vi "ProyectoFinal.vi"() -> ()   [LabVIEW 2020]
uses:
  <vilib>/Instr/_visa.llb/VISA Configure Serial Port (Instr).vi
  <vilib>/addons/control/pid/pid.llb/PID (DBL).vi
  <vilib>/addons/control/pid/NI_PID_pid.lvlib
panel:
  out "Thermometer A":dbl(slide) scale=0.0..32.0
  in  "MANUAL / MATERIAL":bool
  in  "LISTA DE MATERIALES":string(combo)
  out "Temp Reci 2":dbl
  out "Temp Reci":dbl
  in  "EXTRUIR":bool
  out "PRECALENTADO":bool
  in  "Set Point":dbl(slide) scale=0.0..40.0
  out "Temp Fil 2":dbl
  out "ERROR 2":dbl
  out "ErrorPID 2":dbl
  out "Error PID 2":dynamicdata(graph)
  out "Temperatura 2":dynamicdata(graph)
  out "Error PID":dynamicdata(graph)
  in  "VISA resource name":refnum<visa-resource-name>
  in  "stop":bool
  out "ERROR":dbl
  out "Temperatura":dynamicdata(graph)
  out "Temp Fil":dbl
  out "ErrorPID":dbl
  # "CONTROLADOR SISTEMA TERMICO CON CONTROL PID COMUNICACION SERIE"
  # "UNIDAD PROFESIONAL DE INGENIERIA CAMPUS ZACATECAS - INSTITUTO POLITECNICO NACIONAL\nUNIDAD DE APREDIZAJE DE INSTRUMENTACION VIRTUAL\nDIEGO JAUREGUI ONTIVEROS  | CARLOS CASAS CASAS | ALEJANDRO LOPEZ GONZALEZ"
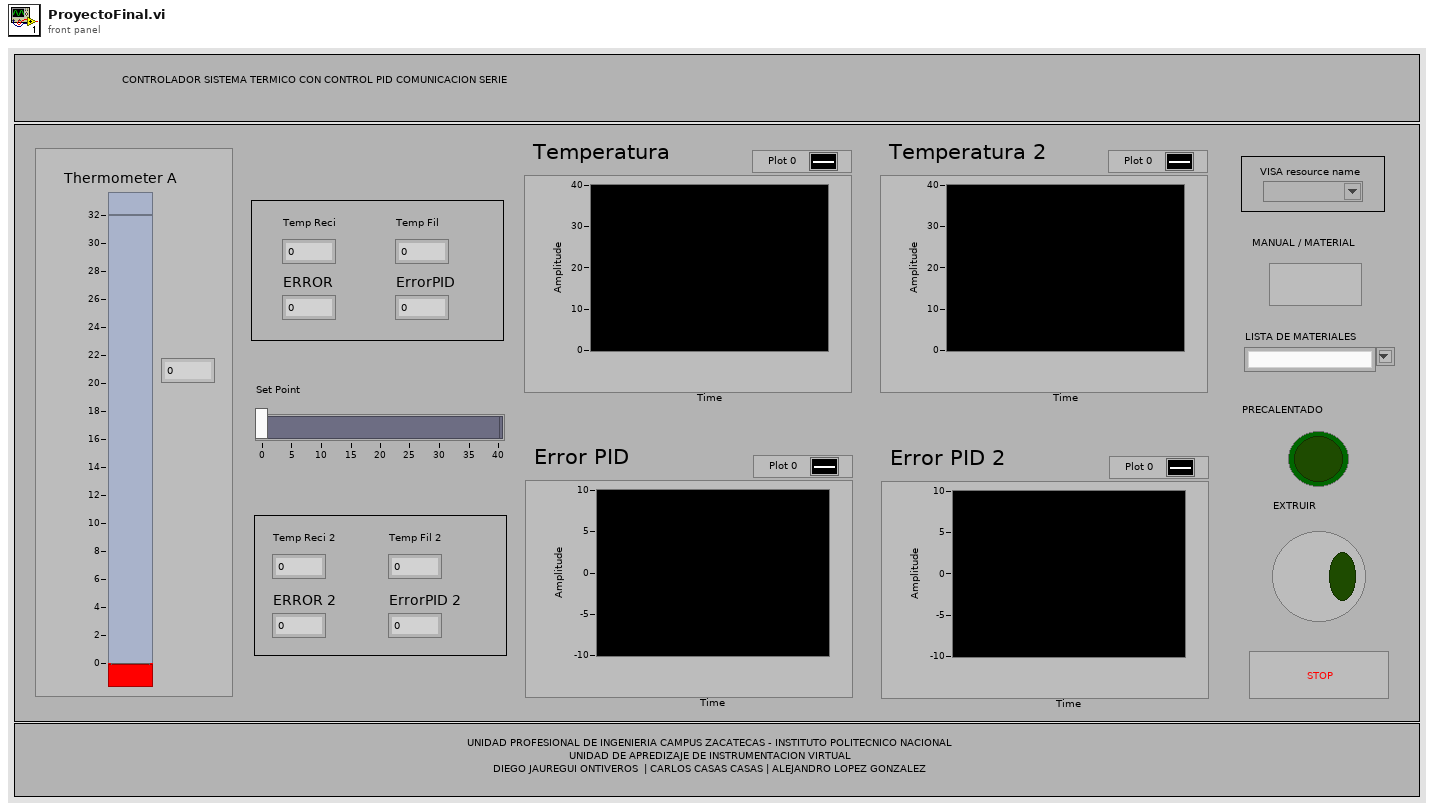
[diagram p1: front panel]
types:
  T1 = cluster{"proportional gain (Kc)":dbl, "integral time (Ti, min)":dbl, "derivative time (Td, min)":dbl}
  T2 = enum8{"Enabled", "Disabled", "Disabled and Grayed Out"}
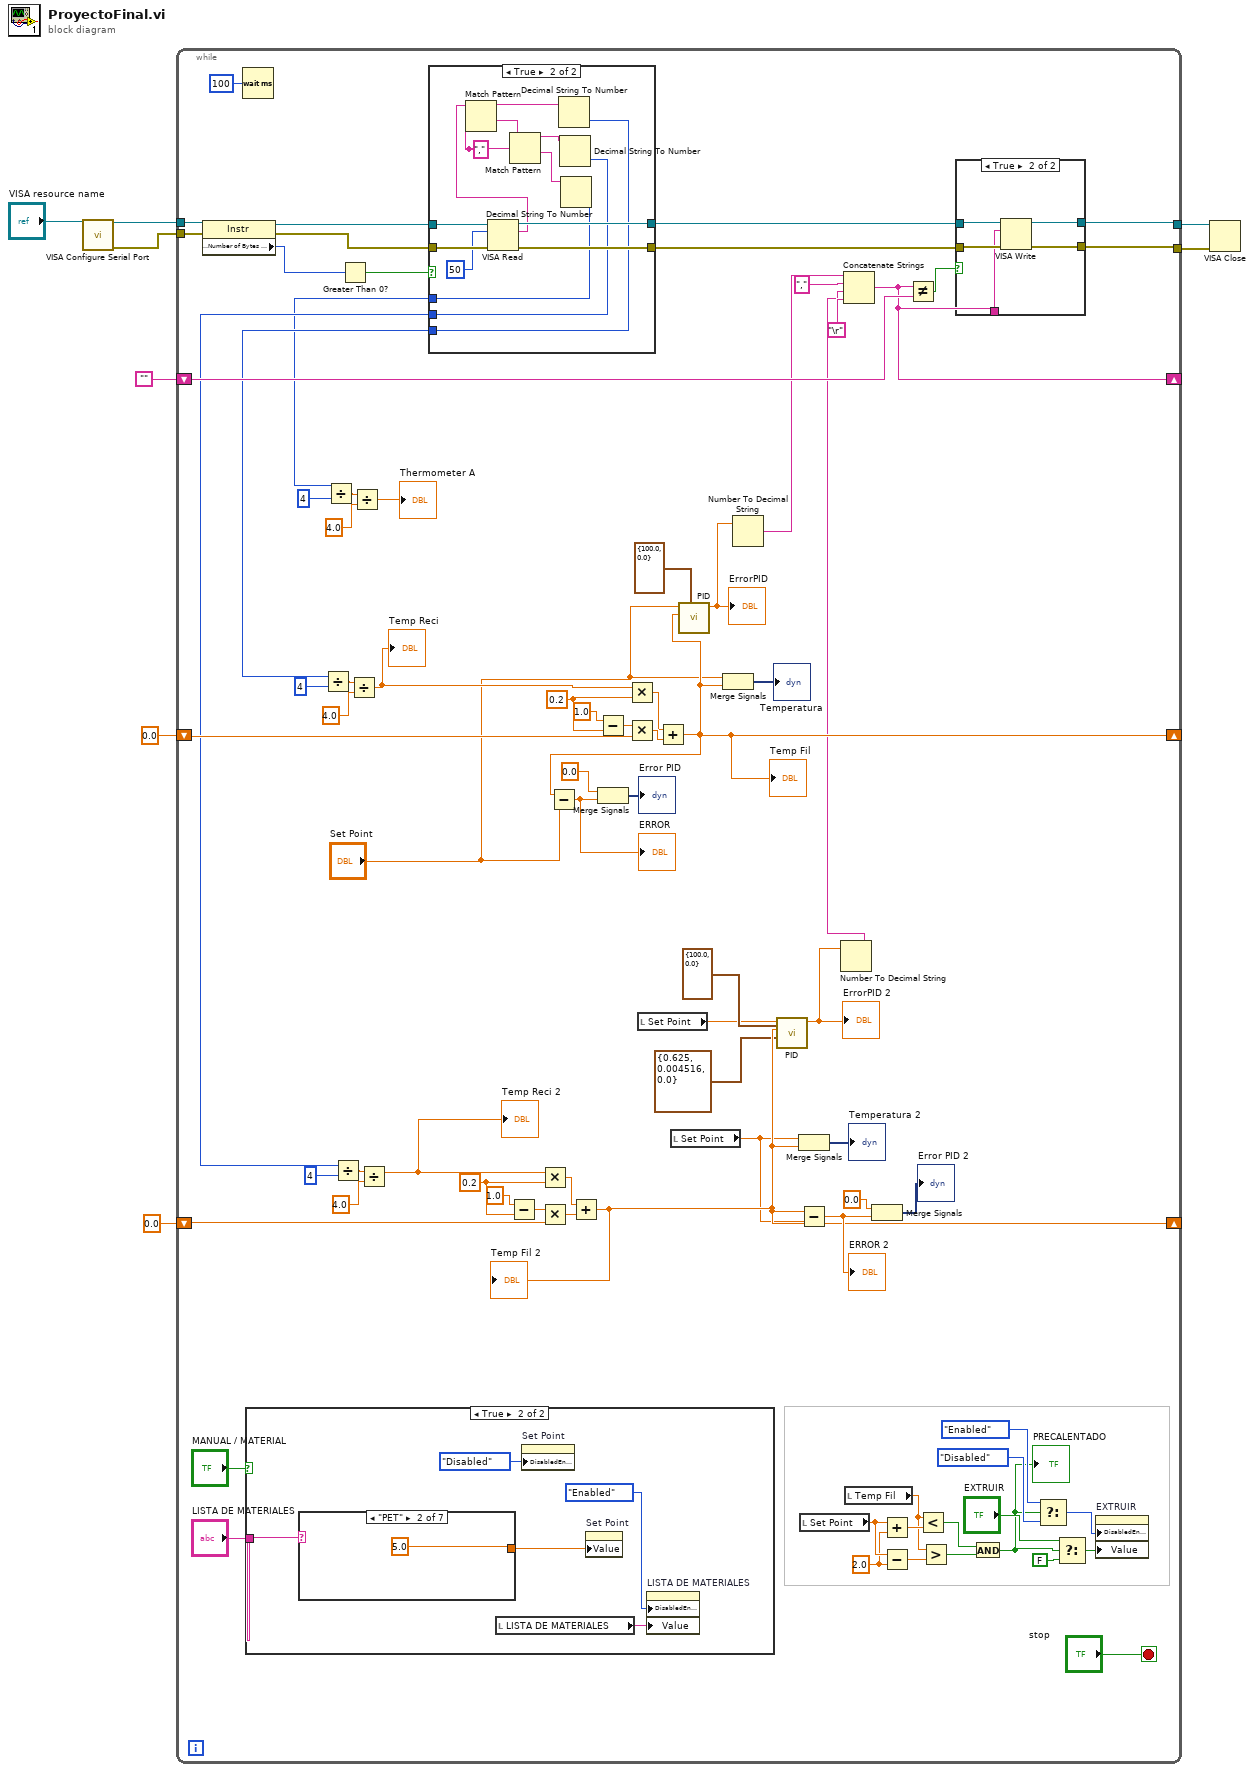
[diagram p0: block diagram]
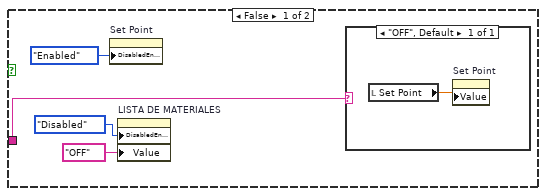
[diagram p2: hidden frame]
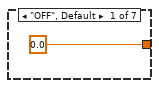
[diagram p3: hidden frame]
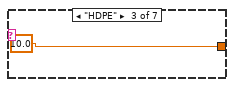
[diagram p4: hidden frame]
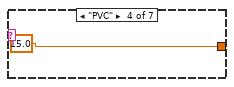
[diagram p5: hidden frame]
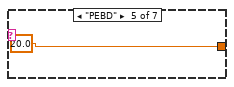
[diagram p6: hidden frame]
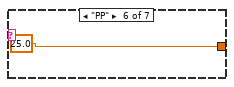
[diagram p7: hidden frame]
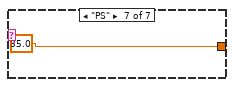
[diagram p8: hidden frame]
diagram:
  n1 = call-poly "VISA Configure Serial Port"("VISA resource name"="VISA resource name") -> ("VISA resource name out"=w6:refnum<visa-resource-name>, "error out"=w5:errorcluster)  [unwired: 13 in]
  n2 = while {
    tunnel: [w87] -> w8
    tunnel: [w86] -> w7
    tunnel: w6 -> [w85]
    tunnel: w5 -> [w84]
    shift-right: [w82] -> _
    shift-left: "" -> [w83]
    shift-right: [w44] -> _
    shift-left: 0.0 -> [w66]
    shift-right: [w12] -> _
    shift-left: 0.0 -> [w49]
    stop <- "stop" stop-if-true
    w29 = 2.0 ("y")
    w52 = 0.2
    w68 = 0.2
    n3 = property class="Instr"(reference=w85, error in=w84) -> (reference out=w80:refnum<visa-resource-name>, error out=w78:errorcluster, "Serial Settings:Number of Bytes at Serial Port"=w75:u32)
    n4 = Wait (ms)(milliseconds to wait=u32 100) -> ()  [unwired: 1 out]
    n5 = case shown="True" "MANUAL / MATERIAL" {
      tunnel: "LISTA DE MATERIALES" -> [w89 w95]
      frame False {
        n6 = property on="Set Point" class="Slide (strict)"("DisabledEnum"=T2."Enabled" ("Disabled")) -> ()  [unwired: 2 in, 2 out]
        n7 = property on="LISTA DE MATERIALES" class="CmbBox"("DisabledEnum"=T2."Disabled" ("Disabled"), "Value"="OFF" ("LISTA DE MATERIALES")) -> ()  [unwired: 2 in, 2 out]
        n8 = case shown="\"OFF\", Default" w89 {
          frame "OFF", Default {
            n9 = local read "Set Point"() -> (w93:dbl)
            n10 = property on="Set Point" class="Slide (strict)"("Value"=w93) -> ()  [unwired: 2 in, 2 out]
          }
        }
      }
      frame True {
        n11 = case shown="\"PET\"" w95 {
          tunnel: [0.0 ("Set Point") 5.0 ("Set Point") 10.0 ("Set Point") 15.0 ("Set Point") 20.0 ("Set Point") 25.0 ("Set Point") 35.0 ("Set Point")] -> w94
          frame "OFF", Default {
          }
          frame "PET" {
          }
          frame "HDPE" {
          }
          frame "PVC" {
          }
          frame "PEBD" {
          }
          frame "PP" {
          }
          frame "PS" {
          }
        }
        n12 = local read "LISTA DE MATERIALES"() -> (w96:string)
        n13 = property on="Set Point" class="Slide (strict)"("DisabledEnum"=T2."Disabled" ("Disabled")) -> ()  [unwired: 2 in, 2 out]
        n14 = property on="Set Point" class="Slide (strict)"("Value"=w94) -> ()  [unwired: 2 in, 2 out]
        n15 = property on="LISTA DE MATERIALES" class="CmbBox"("DisabledEnum"=T2."Enabled" ("Disabled"), "Value"=w96) -> ()  [unwired: 2 in, 2 out]
      }
    }
    n16 = Greater Than 0?(x=w75) -> (x > 0?=w76:bool)
    n17 = case shown="True" w76 {
      tunnel: w80 -> [w107 w121]
      tunnel: [w107 w120] -> w79
      tunnel: w78 -> [w106 w119]
      tunnel: [w106 w118] -> w77
      tunnel: [_ w116] -> w59
      tunnel: [_ w113] -> w45
      tunnel: [_ w108] -> w14
      frame False {
      }
      frame True {
        w111 = "," ("regular expression")
        n18 = VISA Read(VISA resource name=w121, byte count=u32 50, error in (no error)=w119) -> (VISA resource name out=w120:refnum<visa-resource-name>, read buffer=w115:string, error out=w118:errorcluster)  [unwired: 1 out]
        n19 = Match Pattern(string=w115, regular expression=w111) -> (before substring=w114:string, after substring=w112:string)  [unwired: 1 in, 2 out]
        n20 = Match Pattern(string=w112, regular expression=w111) -> (before substring=w110:string, after substring=w109:string)  [unwired: 1 in, 2 out]
        n21 = Decimal String To Number(string=w114) -> (number=w116:i32)  [unwired: 2 in, 1 out]
        n22 = Decimal String To Number(string=w110) -> (number=w113:i32)  [unwired: 2 in, 1 out]
        n23 = Decimal String To Number(string=w109) -> (number=w108:i32)  [unwired: 2 in, 1 out]
      }
    }
    n24 = Divide(x=w59, y=4) -> (x/y=w73:dbl)
    n25 = Divide(x=w14, y=4) -> (x/y=w17:dbl)
    n26 = Divide(x=w45, y=4) -> (x/y=w57:dbl)
    n27 = Divide(x=w73, y=4.0) -> (x/y=w21:dbl)
    "Temp Reci" <- w21
    n28 = Divide(x=w17, y=4.0) -> (x/y=→"Thermometer A":dbl)
    n29 = Divide(x=w57, y=4.0) -> (x/y=w22:dbl)
    "Temp Reci 2" <- w22
    n30 = Subtract(x=1.0, y=w52) -> (x-y=w53:dbl)
    n31 = Multiply(x=w22, y=w52) -> (x*y=w54:dbl)
    n32 = Multiply(x=w53, y=w49) -> (x*y=w55:dbl)
    n33 = Add(x=w54, y=w55) -> (x+y=w12:dbl)
    "Temp Fil 2" <- w12
    n34 = Subtract(x=1.0, y=w68) -> (x-y=w69:dbl)
    n35 = Multiply(x=w21, y=w68) -> (x*y=w70:dbl)
    n36 = Multiply(x=w69, y=w66) -> (x*y=w71:dbl)
    n37 = local read "Set Point"() -> (w11:dbl)
    n38 = Add(x=w70, y=w71) -> (x+y=w44:dbl)
    "Temp Fil" <- w44
    n39 = Subtract(x=w44, y="Set Point") -> (x-y=w61:dbl)
    "ERROR" <- w61
    n40 = Merge Signals(0.0, w61) -> (→"Error PID":dynamicdata)
    n41 = local read "Set Point"() -> (w10:dbl)
    n42 = call-poly <vilib>:"PID.vi"("output range"=cluster{"output high":dbl, "output low":dbl} {"output high"=100.0, "output low"=0.0}, "process variable"=w44, "setpoint"="Set Point") -> ("output"=w43:dbl)  [unwired: 7 in, 1 out]
    "ErrorPID" <- w43
    n43 = Merge Signals("Set Point", w44) -> (→"Temperatura":dynamicdata)
    n44 = Number To Decimal String(number=w43) -> (decimal integer string=w42:string)  [unwired: 1 in]
    n45 = call-poly <vilib>:"PID.vi"("output range"=cluster{"output high":dbl, "output low":dbl} {"output high"=100.0, "output low"=0.0}, "PID gains"=T1 {"proportional gain (Kc)"=0.625, "integral time (Ti, min)"=0.004516, "derivative time (Td, min)"=0.0}, "process variable"=w12, "setpoint"=w11) -> ("output"=w37:dbl)  [unwired: 6 in, 1 out]
    "ErrorPID 2" <- w37
    n46 = Merge Signals(w10, w12) -> (→"Temperatura 2":dynamicdata)
    n47 = Subtract(x=w12, y=w10) -> (x-y=w47:dbl)
    "ERROR 2" <- w47
    n48 = local read "Set Point"() -> (w30:dbl)
    n49 = Number To Decimal String(number=w37) -> (decimal integer string=w38:string)  [unwired: 1 in]
    n50 = Concatenate Strings(w42, "," ("string"), w38, "\r") -> (w82:string)
    n51 = local read "Temp Fil"() -> (w26:dbl)
    n52 = Merge Signals(0.0, w47) -> (→"Error PID 2":dynamicdata)
    n53 = Add(x=w30, y=w29) -> (x+y=w28:dbl)
    n54 = Subtract(x=w30, y=w29) -> (x-y=w27:dbl)
    n55 = Not Equal?(x=w82, y=w83) -> (x != y?=w81:bool)
    n56 = Less?(x=w26, y=w28) -> (x < y?=w25:bool)
    n57 = Greater?(x=w26, y=w27) -> (0:w24:bool)
    n58 = case shown="True" w81 {
      tunnel: w79 -> [w123 w128]
      tunnel: w77 -> [w122 w127]
      tunnel: [w123 w126] -> w87
      tunnel: [w122 w125] -> w86
      tunnel: w82 -> [_ w124]
      frame False {
      }
      frame True {
        n59 = VISA Write(VISA resource name=w128, write buffer=w124, error in (no error)=w127) -> (VISA resource name out=w126:refnum<visa-resource-name>, error out=w125:errorcluster)  [unwired: 1 out]
      }
    }
    n60 = And(x=w25, y=w24) -> (x .and. y?=w23:bool)
    "PRECALENTADO" <- w23
    n61 = Select(t=T2."Enabled" ("Disabled"), s=w23, f=T2."Disabled" ("Disabled")) -> (s? t:f=w36:T2)
    n62 = Select(t="EXTRUIR", s=w23, f=FALSE) -> (s? t:f=w33:bool)
    n63 = property on="EXTRUIR" class="Bool (strict)"("DisabledEnum"=w36, "Value"=w33) -> ()  [unwired: 2 in, 2 out]
  }
  n64 = VISA Close(VISA resource name=w8, error in (no error)=w7) -> ()  [unwired: 1 out]
